vi "LIN EX Master Read.vi"(7 "pData":string, 9 "PID":u8, 10 "LINIndex":u8, 11 "DevHandle":i32) -> (3 "function return":i32, 5 "pData out":string)   [LabVIEW 2010, in "usb2lin_ex.lvlib"]
doc: "int WINAPI LIN_EX_MasterRead(int DevHandle,unsigned char LINIndex,unsigned char PID,unsigned char *pData);"
uses:
  usb2lin_ex.lvlib
  USB2XXX/trunk/USB2XXX/USB2XXX/vs2010/Release/USB2XXX.dll
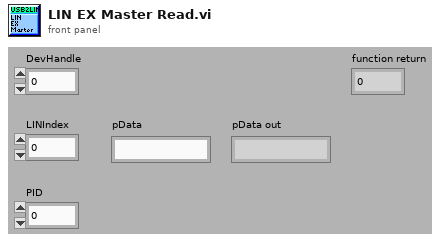
[diagram p1: front panel]
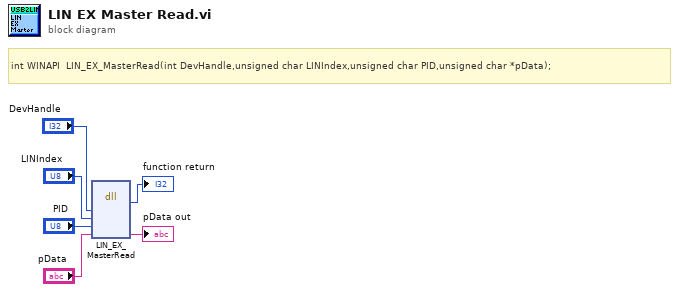
[diagram p0: block diagram]
diagram:
  # "int WINAPI  LIN_EX_MasterRead(int DevHandle,unsigned char LINIndex,unsigned char PID,unsigned char *pData);"
  n1 = dll-call lib="E:/Projects/USB2XXX/trunk/USB2XXX/USB2XXX/vs2010/Release/USB2XXX.*" fn="LIN_EX_MasterRead"("DevHandle"="DevHandle", "LINIndex"="LINIndex", "PID"="PID", "pData"="pData") -> (→"function return":i32, "pData"=→"pData out":string)  [unwired: 6 in, 2 out]
